vi "DC Voltage RMS Measurements.vi"(8 "error in (no error)":errorcluster, 10 "Waveform Data":waveform(dbl), 11 "Instrument Input":refnum<k15>) -> (0 "error out":errorcluster, 1 "RMS value":dbl, 2 "DC value":dbl, 3 "Instrument Output":refnum<k15>)   [LabVIEW 2024, in "NIDmmDCRmsVoltage.lvlib"]
uses:
  NIDmmDCRmsVoltage.lvlib
  <vilib>/measure/NI_MAPro.lvlib
  <vilib>/measure/madcrms.llb/Basic Averaged DC-RMS for 1 Chan.vi
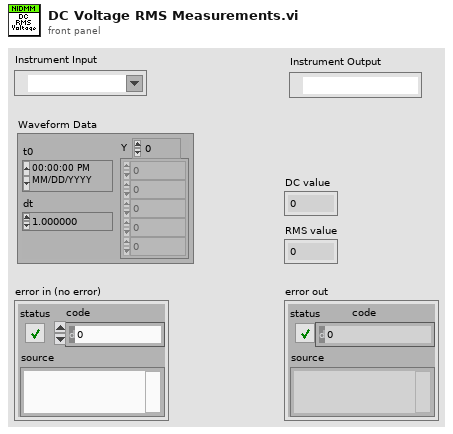
[diagram p1: front panel]
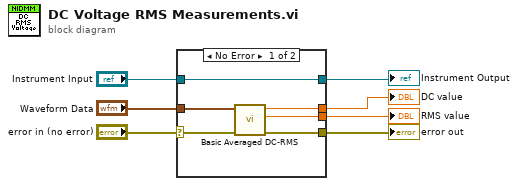
[diagram p0: block diagram]
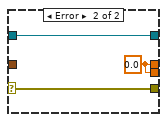
[diagram p2: hidden frame]
diagram:
  n1 = case shown="No Error" "error in (no error)" {
    selector: "error in (no error)" -> [w8 w16]
    tunnel: "Waveform Data" -> [w13 _]
    tunnel: [w12 w14] -> w6
    tunnel: [w11 w14] -> w5
    tunnel: [w10 w16] -> w4
    tunnel: "Instrument Input" -> [w9 w15]
    tunnel: [w9 w15] -> w1
    frame No Error {
      n2 = call-poly <vilib>:"Basic Averaged DC-RMS.vi"("error in (no error)"=w8, "signal in"=w13) -> ("error out"=w10:errorcluster, "RMS value"=w12:dbl, "DC value"=w11:dbl)  [unwired: 6 in, 1 out]
    }
    frame Error {
      w14 = 0.0 ("DC value")
    }
  }
  "RMS value" <- w6
  "DC value" <- w5
  "error out" <- w4
  "Instrument Output" <- w1
